vi "XCorLocalize.vi"(1 "GPU Image Pointer":u64, 2 "InitialPos":cluster{"X":dbl, "Y":dbl}) -> (0 "position":cluster{"X":dbl, "Y":dbl})   [LabVIEW 2011]
uses:
  cudatrack-debug.dll
panel:
  in  "Output position":cluster{"X":dbl, "Y":dbl}
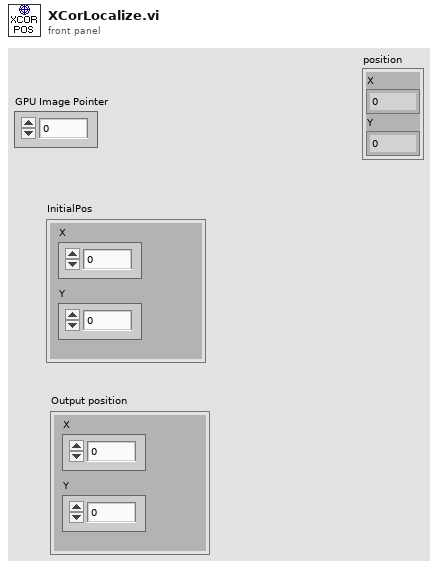
[diagram p1: front panel]
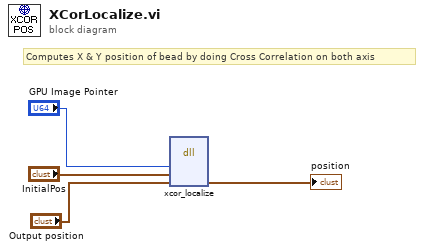
[diagram p0: block diagram]
diagram:
  # "Computes X & Y position of bead by doing Cross Correlation on both axis"
  n1 = dll-call lib="D:/jcnossen1/cudaqi-tracker/cudaqi/cudatrack-debug.dll" fn="xcor_localize"("gpuImage"="GPU Image Pointer", "initialPos"="InitialPos", "position"="Output position") -> ("position"=→"position":cluster{"X":dbl, "Y":dbl})  [unwired: 6 in, 2 out]
